vi "FileIO-Delete Files.vi"(0 "Folder":path, 9 "Pattern":string, 11 "error in (no error)":errorcluster) -> (15 "error out":errorcluster)   [LabVIEW 2020]
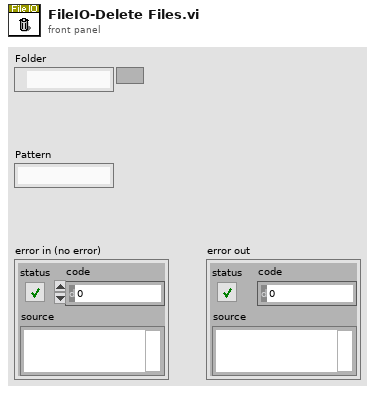
[diagram p1: front panel]
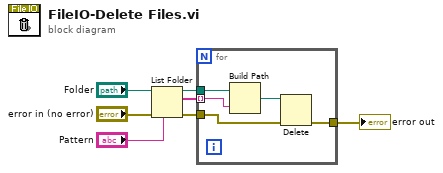
[diagram p0: block diagram]
diagram:
  n1 = List Folder(path="Folder", pattern="Pattern", error in="error in (no error)") -> (path out=w2:path, filenames=w3:string[], error out=w4:errorcluster)  [unwired: 1 in, 1 out]
  n2 = for {
    tunnel: w2 -> [w12]
    tunnel: w3 -> [w11] mode=indexing
    tunnel: w4 -> [w9]
    tunnel: [w8] -> w5
    n3 = Build Path(base path=w12, name or relative path=w11) -> (appended path=w10:path)
    n4 = Delete(path (use dialog)=w10, error in=w9) -> (error out=w8:errorcluster)  [unwired: 3 in, 2 out]
  }
  "error out" <- w5
